vi "Read Configuration.vi"(8 "error in (no error)":errorcluster, 11 "Motor Base in":refnum<class "Motor Base.lvclass">) -> (0 "error out":errorcluster, 2 "Configuration":T1={"Modes of operation"=8, "Feed(pulse)"=1000000, "Max motor speed(r/min)"=200, "Max torque(0.1%)"=500, "Min position limit(pulse)"=-2147483648, "Max position limit(pulse)"=2147483647} {"Modes of operation" items=["No mode change/no mode assigned"=0, "Profile position mode"=1, "Velocity mode"=2, "Profile velocity mode"=3, "Torque profile mode"=4, "Homing mode"=6, "Interpolated position mode"=7, "Cyclic synchronous position mode"=8, "Cyclic synchronous velocity mode"=9, "Cyclic synchronous torque mode"=10]}, 3 "Motor Base out":refnum<class "Motor Base.lvclass">)   [LabVIEW 2016, in "Motor Base.lvlib" / "Motor Base.lvclass"]
uses:
  Motor Base.lvclass
  Motor Base.lvclass/Motor Base.ctl
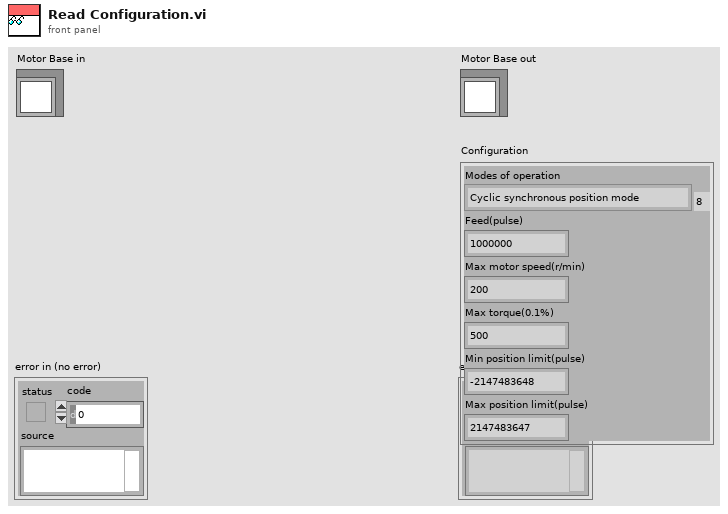
[diagram p1: front panel]
types:
  T1 = cluster{"Modes of operation":i8, "Feed(pulse)":u32, "Max motor speed(r/min)":u32, "Max torque(0.1%)":u16, "Min position limit(pulse)":i32, "Max position limit(pulse)":i32}
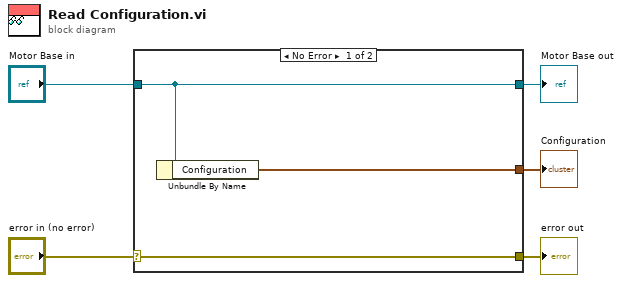
[diagram p0: block diagram]
diagram:
  n1 = case shown="No Error" "error in (no error)" {
    selector: "error in (no error)" -> [w8 w9]
    tunnel: [w8 w9] -> w4
    tunnel: [w7 w10] -> w2
    tunnel: "Motor Base in" -> [w7 w10]
    tunnel: [w6 _] -> w1
    frame No Error {
      n2 = Unbundle By Name(w7) -> ("Configuration"=w6:T1)
    }
    frame Error {
    }
  }
  "error out" <- w4
  "Motor Base out" <- w2
  "Configuration" <- w1
